vi "ReadData.vi"() -> ()   [LabVIEW 2020]
uses:
  <vilib>/addons/database/_DB Variant To Data/Database Variant To Data.xnode
  <vilib>/addons/database/NI_Database_API.lvlib
panel:
  out "Results":string
  out "data1":variant[][](array[variant])
  out "error out":errorcluster
  in  "error in (no error)":errorcluster
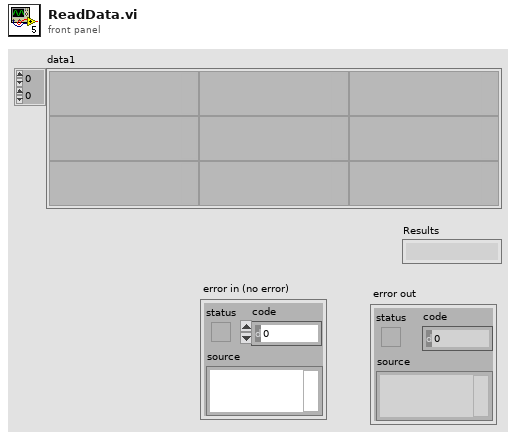
[diagram p1: front panel]
types:
  T1 = typedef "NI_Database_API.lvlib/Conn ObjectReference.ctl" = refnum<k1>
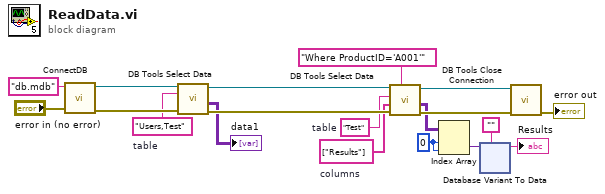
[diagram p0: block diagram]
diagram:
  w4 = 0 ("index (row)")
  w7 = "Test"  # table
  w10 = string[] ["Results"]  # columns
  w11 = "Users,Test"  # table
  n1 = call "ConnectDB.vi"("error in (no error)"="error in (no error)", "Filename"="db.mdb") -> ("error out"=w16:errorcluster, "DB Conn"=w17:T1)  [unwired: 8 in]
  n2 = call <vilib>:"DB Tools Select Data.vi"("error in (no error)"=w16, "table"=w11, "connection reference"=w17) -> ("error out"=w15:errorcluster, "data"=→"data1":variant[][], "connection reference out"=w14:T1)  [unwired: 3 in]
  n3 = call <vilib>:"DB Tools Select Data.vi"("condition"="Where ProductID='A001'", "error in (no error)"=w15, "columns"=w10, "table"=w7, "connection reference"=w14) -> ("error out"=w12:errorcluster, "data"=w5:variant[][], "connection reference out"=w13:T1)  [unwired: 1 in]
  n4 = Index Array(array=w5, index (row)=w4, index (col)=w4) -> (element=w3:variant)
  n5 = xnode "Database Variant To Data"("database variant"=w3, "type"="") -> ("data"=→"Results":string)  [unwired: 1 in, 1 out]
  n6 = call <vilib>:"DB Tools Close Connection.vi"("error in (no error)"=w12, "connection reference"=w13) -> ("error out"=→"error out":errorcluster)  [unwired: 5 in]
